vi "Read Setpoint Settings.vi"(7 "listen period":sgl=0.1, 8 "error in":errorcluster, 11 "Brooks MFC in":refnum<class "Brooks MFC.lvclass">) -> (0 "error out":errorcluster, 2 "Setpoint Settings":T1={"Analog Setpoint Span"=0.997014, "Analog Setpoint Offset"=-0.314216, "Softstart Ramp Value"=100.0, "Setpoint Source"=3, "Softstart Type"=0} {"Softstart Type" items=["Softstart disabled", "Non-linear softstart", "Linear up only softstart", "Linear down only softstart", "Linear up and down softstart", "Undefined"]; "Setpoint Source" items=["Undefined", "0..5 volt or 0..20mA input", "1..5 volt or 4..20mA input", "Communication input"]}, 3 "Brooks MFC out":refnum<class "Brooks MFC.lvclass">)   [LabVIEW 2016, in "Brooks MFC.lvclass"]
uses:
  Brooks MFC.lvclass
  Setpoint Settings.ctl
  Brooks MFC.lvclass/Brooks MFC.ctl
  Instance           3 30Saved   Read Setpoint Settings .vi
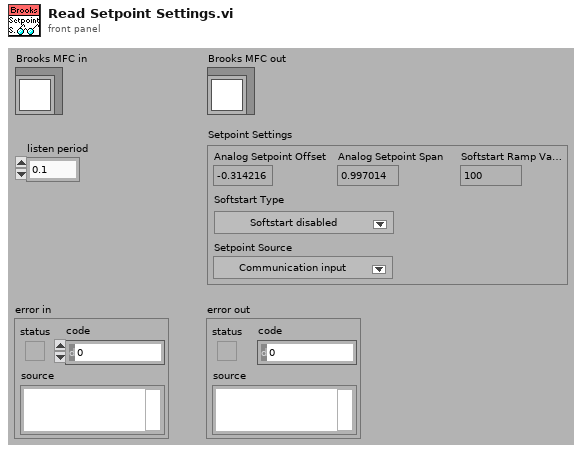
[diagram p1: front panel]
types:
  T1 = typedef "Brooks MFC.lvclass/Setpoint Settings.ctl" = cluster{"Analog Setpoint Span":sgl, "Analog Setpoint Offset":sgl, "Softstart Ramp Value":sgl, "Setpoint Source":u8, "Softstart Type":u8}
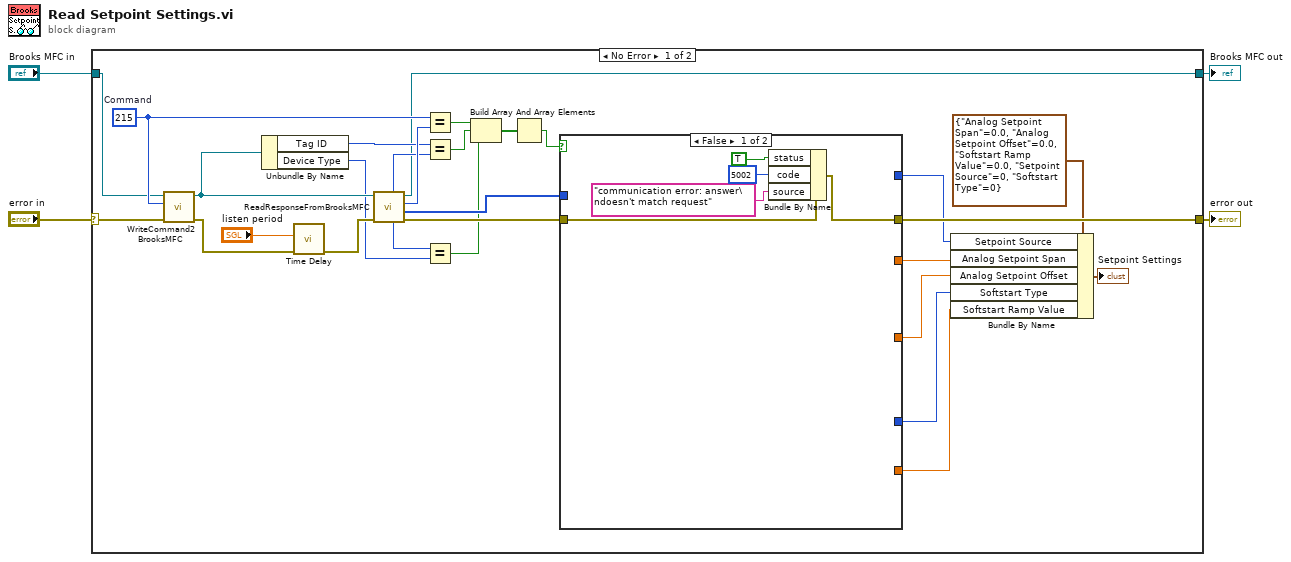
[diagram p0: block diagram]
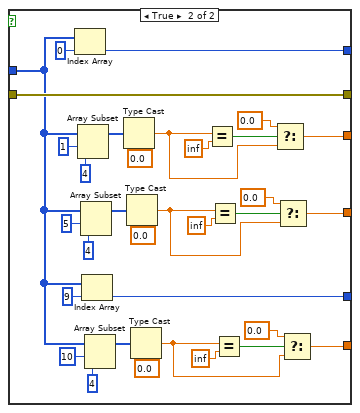
[diagram p2: hidden frame]
diagram:
  n1 = case shown="No Error" "error in" {
    selector: "error in" -> [w14 w71]
    tunnel: "Brooks MFC in" -> [w15 w72]
    tunnel: [w13 w72] -> w2
    tunnel: [w12 w71] -> w1
    frame No Error {
      w19 = u8 215  # Command
      n2 = call "WriteCommand2BrooksMFC.vi"("error in"=w14, "Command"=w19, "Brooks MFC in"=w15) -> ("error out"=w29:errorcluster, "Brooks MFC out"=w18:refnum<class "Brooks MFC.lvclass">)  [unwired: 6 in, 1 out]
      n3 = Unbundle By Name(w18) -> ("Tag ID"=w16:u32, "Device Type"=w17:u8)
      n4 = call "Time Delay"("error in (no error)"=w29, "Delay Time (s)"="listen period") -> ("error out"=w27:errorcluster)  [unwired: 9 in]
      n5 = call "ReadResponseFromBrooksMFC.vi"("error in"=w27, "Brooks MFC in"=w18) -> ("error out"=w32:errorcluster, "Data"=w31:u8[], "Command"=w30:u8, "Brooks MFC out"=w13:refnum<class "Brooks MFC.lvclass">, "device type"=w25:u8, "tag ID"=w26:u32)  [unwired: 4 in]
      n6 = Equal?(x=w19, y=w30) -> (x = y?=w24:bool)
      n7 = Equal?(x=w16, y=w26) -> (x = y?=w23:bool)
      n8 = Equal?(x=w25, y=w17) -> (x = y?=w22:bool)
      n9 = Build Array(w24, w23, w22) -> (w21:bool[])
      n10 = And Array Elements(Boolean array=w21) -> (logical AND=w20:bool)
      n11 = case shown="False" w20 {
        tunnel: w31 -> [_ w42]
        tunnel: w32 -> [w35 w68]
        tunnel: [w34 w68] -> w12
        tunnel: [_ w64] -> w9
        tunnel: [_ w51] -> w8
        tunnel: [_ w40] -> w7
        tunnel: [_ w39] -> w6
        tunnel: [_ w38] -> w10
        frame False {
          n12 = Bundle By Name(cluster=w35, "status"=TRUE ("Bundle Element"), "code"=5002 ("Bundle Element"), "source"="communication error: answer\ndoesn't match request") -> (w34:errorcluster)
        }
        frame True {
          n13 = Index Array(array=w42, index=0 ("Index")) -> (element=w38:u8)
          n14 = Array Subset(array=w42, index=1 ("Array Index"), length=4 ("Array Length")) -> (w63:u8[])
          n15 = Array Subset(array=w42, index=5 ("Array Index"), length=4 ("Array Length")) -> (w55:u8[])
          n16 = Index Array(array=w42, index=9 ("Index")) -> (element=w39:u8)
          n17 = Array Subset(array=w42, index=10 ("Array Index"), length=4 ("Array Length")) -> (w45:u8[])
          n18 = Type Cast(type=sgl 0.0 ("x"), x=w63) -> (*(type *) &x=w61:sgl)
          n19 = Type Cast(type=sgl 0.0 ("x"), x=w55) -> (*(type *) &x=w53:sgl)
          n20 = Type Cast(type=sgl 0.0 ("x"), x=w45) -> (*(type *) &x=w41:sgl)
          n21 = Equal?(x=w61, y=sgl inf ("Single")) -> (x = y?=w66:bool)
          n22 = Equal?(x=w53, y=sgl inf ("Single")) -> (x = y?=w57:bool)
          n23 = Equal?(x=w41, y=sgl inf ("Single")) -> (x = y?=w47:bool)
          n24 = Select(t=sgl 0.0 ("x"), s=w66, f=w61) -> (s? t:f=w64:sgl)
          n25 = Select(t=sgl 0.0 ("x"), s=w57, f=w53) -> (s? t:f=w51:sgl)
          n26 = Select(t=sgl 0.0 ("x"), s=w47, f=w41) -> (s? t:f=w40:sgl)
        }
      }
      n27 = Bundle By Name(cluster=T1 {"Analog Setpoint Span"=0.0, "Analog Setpoint Offset"=0.0, "Softstart Ramp Value"=0.0, "Setpoint Source"=0, "Softstart Type"=0} ("Setpoint Settings"), "Setpoint Source"=w10, "Analog Setpoint Span"=w9, "Analog Setpoint Offset"=w8, "Softstart Type"=w6, "Softstart Ramp Value"=w7) -> (→"Setpoint Settings":T1)
    }
    frame Error {
    }
  }
  "Brooks MFC out" <- w2
  "error out" <- w1
